vi "RunOperation.vi"(10 "Inputs":string[](array[string]), 11 "CoreOperation in":refnum<class "CoreOperation.lvclass">) -> (1 "Output/Failure":string, 2 "CLI Process Return Code":i32, 3 "CoreOperation out":refnum<class "CoreOperation.lvclass">)   [LabVIEW 2014, in "CoreOperation.lvclass"]
uses:
  CoreOperation.lvclass
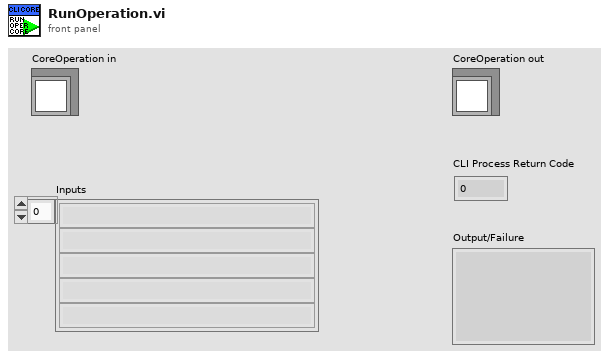
[diagram p1: front panel]
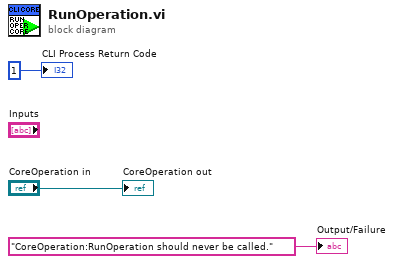
[diagram p0: block diagram]
diagram:
  "CoreOperation out" <- "CoreOperation in"
  "CLI Process Return Code" <- 1 ("CLI Process Return Code")
  "Output/Failure" <- "CoreOperation:RunOperation should never be called." ("Output/Failure")
